vi "Configure User Delay.vi"(6 "Delay Time (0 sec)":dbl min=0.0 max=1000.0, 7 "Delay (T: Auto)":bool, 8 "error in (no error)":errorcluster, 9 "User Delay (1)":i32 min=1 max=5 step=1, 11 "VISA resource name":refnum<visa-resource-name>) -> (0 "error out":errorcluster, 3 "VISA resource name out":refnum<visa-resource-name>)   [LabVIEW 2009, in "Keithley DMM7510.lvlib"]
doc: "This VI enables or disables the automatic delay that occurs before each measurement. This also sets a user-defined delay that you can use in the trigger model."
uses:
  Keithley DMM7510.lvlib
panel:
  in  "Function":u16(ring) items=["Voltage: DC", "Voltage: AC", "Current: DC", "Current: AC", "2W Resistance", "4W Resistance", "Diode", "Capacitance", "Temperature", "Continuity", "Frequency", "Period", "Ratio", "Digitize Voltage", "Digitize Current"]
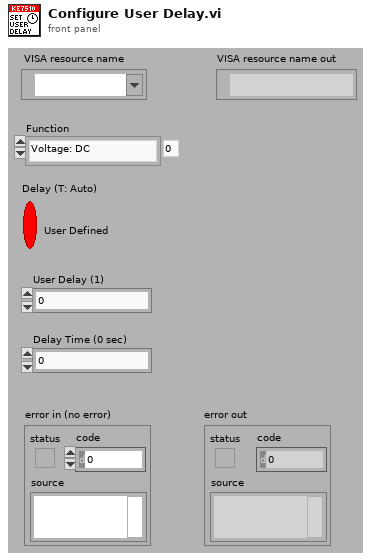
[diagram p1: front panel]
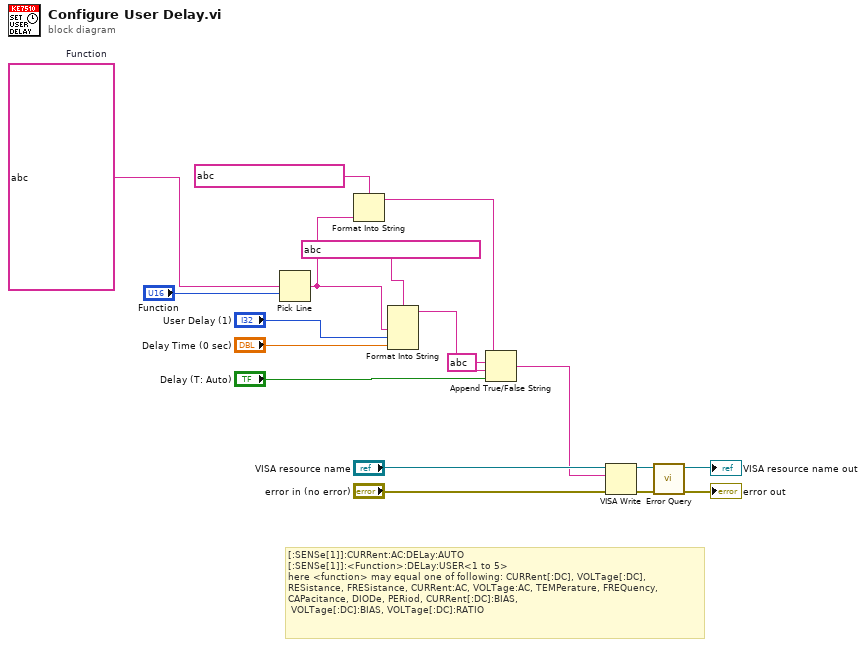
[diagram p0: block diagram]
diagram:
  w5 = string ?  # Function
  # "[:SENSe[1]]:CURRent:AC:DELay:AUTO\n[:SENSe[1]]:<Function>:DELay:USER<1 to 5> \nhere <function> may equal one of following: CURRent[:DC], VOLTage[:DC], \nRESistance, FRESistance, CURRent:AC, VOLTage:AC, TEMPerature, FREQuency, \nCAPacitance, DIODe, PERiod, CURRent[:DC]:BIAS,\n VOLTage[:DC]:BIAS, VOLTage[:DC]:RATIO"
  n1 = Pick Line(multi-line string=w5, line index="Function") -> (output string=w3:string)  [unwired: 1 out]
  n2 = Format Into String(format string=string ?, w3) -> (resulting string=w2:string)  [unwired: 2 in, 1 out]
  n3 = Format Into String(format string=string ?, w3, "User Delay (1)", "Delay Time (0 sec)") -> (resulting string=w9:string)  [unwired: 2 in, 1 out]
  n4 = Append True/False String(1:"Delay (T: Auto)", 2:w9, 3:string ? ("true string"), 4:w2) -> (0:w8:string)
  n5 = VISA Write(VISA resource name="VISA resource name", write buffer=w8, error in (no error)="error in (no error)") -> (VISA resource name out=w16:refnum<visa-resource-name>, error out=w15:errorcluster)  [unwired: 1 out]
  n6 = call "Error Query.vi"("error in (no error)"=w15, "VISA resource name"=w16) -> ("error out"=→"error out":errorcluster, "VISA resource name out"=→"VISA resource name out":refnum<visa-resource-name>)  [unwired: 8 out]
